vi "RegisterNBitSwitchIDInOut.vi"(4 "Switch Bit":bool=TRUE, 6 "N Bit":u16=10, 7 "error in (no error)":errorcluster, 10 "connection ID":refnum<k5>) -> (0 "error out":errorcluster, 3 "connection ID out":refnum<k5>)   [LabVIEW 2012]
panel:
  in  "Register Number":u16=4
  out "Register Swapped":u32=1078
  out "Register swap":dbl[](array[numeric])=[0.0, 1.0, 1.0, 0.0, 1.0, 1.0, 0.0, 0.0, 0.0, 0.0, 1.0, 0.0, 0.0, 0.0, 0.0, 0.0, 0.0, 0.0, 0.0, 0.0, 0.0, 0.0, 0.0, 0.0, 0.0, 0.0, 0.0, 0.0, 0.0, 0.0, 0.0, 0.0]
  out "Register Read":dbl[](array[numeric])=[0.0, 1.0, 1.0, 0.0, 1.0, 1.0, 0.0, 0.0, 0.0, 0.0, 1.0, 0.0, 0.0, 0.0, 0.0, 0.0, 0.0, 0.0, 0.0, 0.0, 0.0, 0.0, 0.0, 0.0, 0.0, 0.0, 0.0, 0.0, 0.0, 0.0, 0.0, 0.0]
  out "Register read":u32=1078
  in  "Device":u16(ring)=4 items=["Attenuation", "Clipping", "Enable channel", "Delay line", "ASIC"]
  # "0     1     2     3     4    5     6     7     8    9    10   11  12   13   14   15"
  # "0     1     2     3     4    5     6     7     8    9    10   11  12   13   14   15"
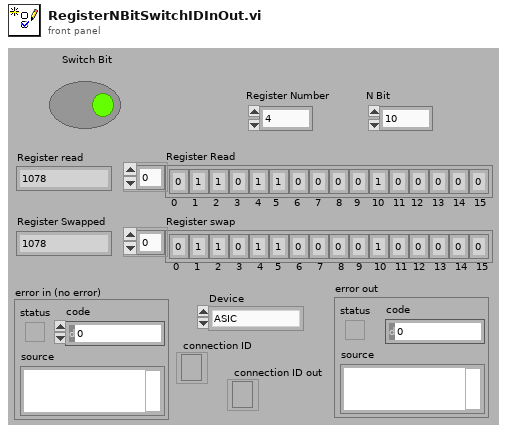
[diagram p1: front panel]
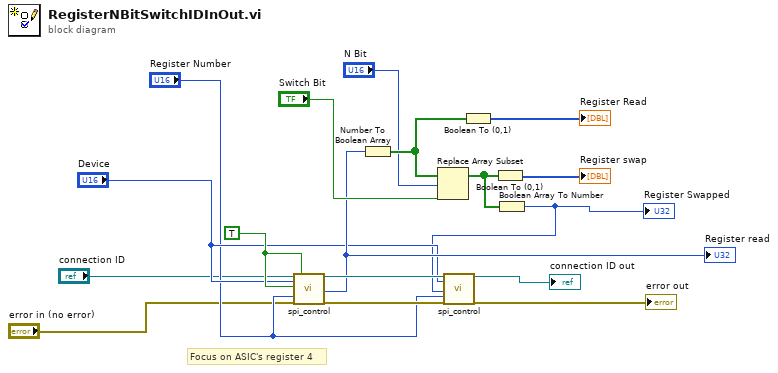
[diagram p0: block diagram]
diagram:
  w10 = TRUE
  # "Focus on ASIC's register 4"
  n1 = call "spi_control.vi"("connection ID"="connection ID", "Device"="Device", "Read/#write"=w10, "Register or channel"="Register Number", "error in"="error in (no error)", "Read physical"=w10) -> ("connection ID out"=w11:refnum<k5>, "data read value"=w9:u32, "error out 2"=w12:errorcluster)  [unwired: 6 in, 5 out]
  "Register read" <- w9
  n2 = Number To Boolean Array(number=w9) -> (Boolean array=w16:bool[])
  n3 = Replace Array Subset(array=w16, new element="Switch Bit", index="N Bit") -> (w13:bool[])
  n4 = Boolean To (0,1)(Boolean=w16) -> (0, 1=→"Register Read":i16[])
  n5 = Boolean To (0,1)(Boolean=w13) -> (0, 1=→"Register swap":i16[])
  n6 = Boolean Array To Number(Boolean array=w13) -> (number=w5:u32)
  "Register Swapped" <- w5
  n7 = call "spi_control.vi"("connection ID"=w11, "Device"="Device", "Data"=w5, "Register or channel"="Register Number", "error in"=w12) -> ("connection ID out"=→"connection ID out":refnum<k5>, "error out 2"=→"error out":errorcluster)  [unwired: 7 in, 6 out]
